vi "Update Position.vi"(8 "error in (no error)":errorcluster, 10 "Current":T1, 11 "Map In":refnum<class "Maze.lvclass">) -> (0 "error out":errorcluster, 1 "At Start?":bool, 2 "Next":T1, 3 "Map Out":refnum<class "Maze.lvclass">)   [LabVIEW 2020, in "Maze.lvclass"]
uses:
  Maze.lvclass
  Position.ctl
  Maze.lvclass/Maze.ctl
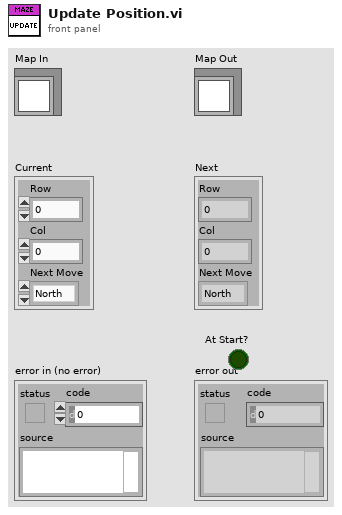
[diagram p1: front panel]
types:
  T1 = typedef "Maze.lvclass/Position.ctl" = cluster{"Row":u64, "Col":u64, "Next Move":enum16{"North", "East", "South", "West", "Halt"}}
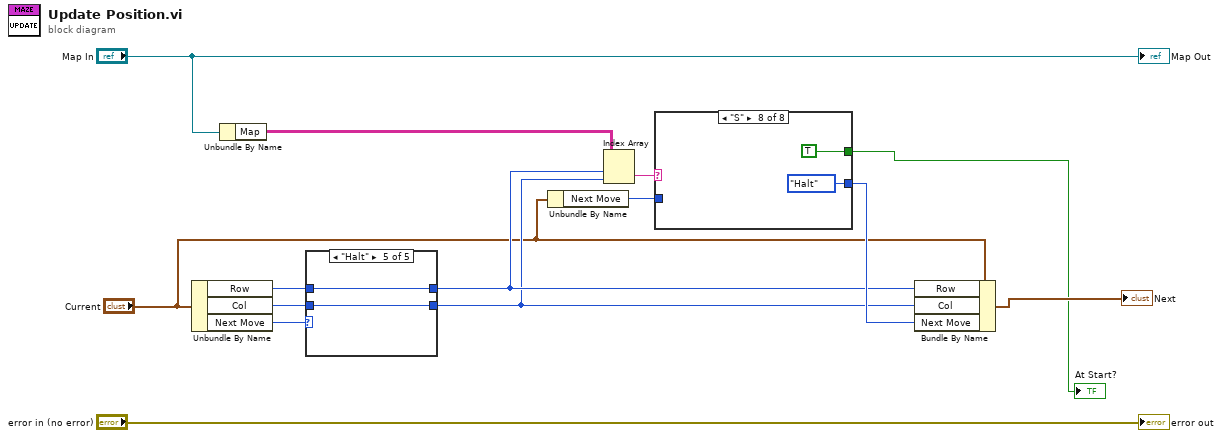
[diagram p0: block diagram]
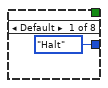
[diagram p2: hidden frame]
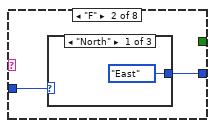
[diagram p3: hidden frame]
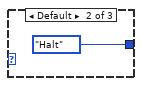
[diagram p4: hidden frame]
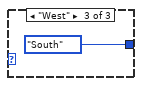
[diagram p5: hidden frame]
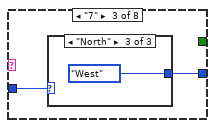
[diagram p6: hidden frame]
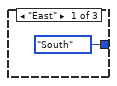
[diagram p7: hidden frame]
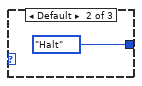
[diagram p8: hidden frame]
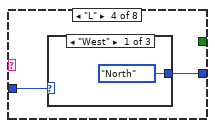
[diagram p9: hidden frame]
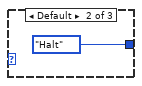
[diagram p10: hidden frame]
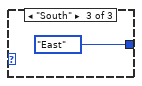
[diagram p11: hidden frame]
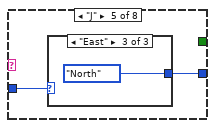
[diagram p12: hidden frame]
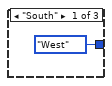
[diagram p13: hidden frame]
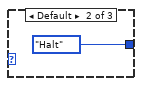
[diagram p14: hidden frame]
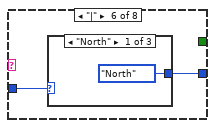
[diagram p15: hidden frame]
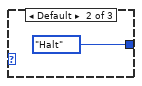
[diagram p16: hidden frame]
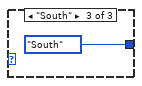
[diagram p17: hidden frame]
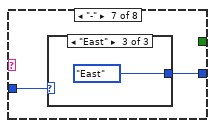
[diagram p18: hidden frame]
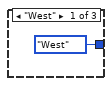
[diagram p19: hidden frame]
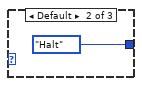
[diagram p20: hidden frame]
diagram:
  n1 = Unbundle By Name("Current") -> ("Row"=w11:u64, "Col"=w10:u64, "Next Move"=w12:enum16{"North", "East", "South", "West", "Halt"})
  n2 = Unbundle By Name("Map In") -> ("Map"=w7:string[][])
  n3 = case shown="\"Halt\"" w12 {
    tunnel: w11 -> [w15 w19 w22 w25 w28]
    tunnel: w10 -> [w17 w20 w23 w26 w27]
    tunnel: [w16 w20 w21 w26 w27] -> w5
    tunnel: [w15 w18 w22 w24 w28] -> w6
    frame "East" {
      n4 = Increment(x=w17) -> (x+1=w16:u64)
    }
    frame "South" {
      n5 = Increment(x=w19) -> (x+1=w18:u64)
    }
    frame "West" {
      n6 = Decrement(x=w23) -> (x-1=w21:u64)
    }
    frame "North" {
      n7 = Decrement(x=w25) -> (x-1=w24:u64)
    }
    frame "Halt" {
    }
  }
  n8 = Unbundle By Name("Current") -> ("Next Move"=w2:enum16{"North", "East", "South", "West", "Halt"})
  n9 = Index Array(array=w7, index (row)=w6, index (col)=w5) -> (element=w4:string)
  n10 = case shown="\"S\"" w4 {
    tunnel: [enum16{"North", "East", "South", "West", "Halt"}."Halt" ("Next Move") w31 w36 w41 w46 w51 w56 enum16{"North", "East", "South", "West", "Halt"}."Halt" ("Next Move")] -> w8
    tunnel: w2 -> [_ w30 w35 w40 w45 w50 w55 _]
    tunnel: [_ _ _ _ _ _ _ TRUE] -> w1
    frame Default {
    }
    frame "F" {
      n11 = case shown="\"North\"" w30 {
        tunnel: [enum16{"North", "East", "South", "West"}."East" ("Next Move") enum16{"North", "East", "South", "West", "Halt"}."Halt" ("Next Move") enum16{"North", "East", "South", "West"}."South" ("Next Move")] -> w31
        frame "North" {
        }
        frame Default {
        }
        frame "West" {
        }
      }
    }
    frame "7" {
      n12 = case shown="\"North\"" w35 {
        tunnel: [enum16{"North", "East", "South", "West"}."South" ("Next Move") enum16{"North", "East", "South", "West", "Halt"}."Halt" ("Next Move") enum16{"North", "East", "South", "West"}."West" ("Next Move")] -> w36
        frame "East" {
        }
        frame Default {
        }
        frame "North" {
        }
      }
    }
    frame "L" {
      n13 = case shown="\"West\"" w40 {
        tunnel: [enum16{"North", "East", "South", "West"}."North" ("Next Move") enum16{"North", "East", "South", "West", "Halt"}."Halt" ("Next Move") enum16{"North", "East", "South", "West"}."East" ("Next Move")] -> w41
        frame "West" {
        }
        frame Default {
        }
        frame "South" {
        }
      }
    }
    frame "J" {
      n14 = case shown="\"East\"" w45 {
        tunnel: [enum16{"North", "East", "South", "West"}."West" ("Next Move") enum16{"North", "East", "South", "West", "Halt"}."Halt" ("Next Move") enum16{"North", "East", "South", "West"}."North" ("Next Move")] -> w46
        frame "South" {
        }
        frame Default {
        }
        frame "East" {
        }
      }
    }
    frame "|" {
      n15 = case shown="\"North\"" w50 {
        tunnel: [enum16{"North", "East", "South", "West"}."North" ("Next Move") enum16{"North", "East", "South", "West", "Halt"}."Halt" ("Next Move") enum16{"North", "East", "South", "West"}."South" ("Next Move")] -> w51
        frame "North" {
        }
        frame Default {
        }
        frame "South" {
        }
      }
    }
    frame "-" {
      n16 = case shown="\"East\"" w55 {
        tunnel: [enum16{"North", "East", "South", "West"}."West" ("Next Move") enum16{"North", "East", "South", "West", "Halt"}."Halt" ("Next Move") enum16{"North", "East", "South", "West"}."East" ("Next Move")] -> w56
        frame "West" {
        }
        frame Default {
        }
        frame "East" {
        }
      }
    }
    frame "S" {
    }
  }
  "At Start?" <- w1
  n17 = Bundle By Name(cluster="Current", "Row"=w6, "Col"=w5, "Next Move"=w8) -> (→"Next":T1)
  "error out" <- "error in (no error)"
  "Map Out" <- "Map In"
